vi "NIDCPower_channel_ganging - configure source mode.vi"(8 "error in (no error)":errorcluster, 9 "source mode":T1=1020 items=["Single Point"=1020, "Sequence"=1021], 11 "Ganged Session In":T2) -> (0 "error out":errorcluster, 3 "Ganged Session Out":T2)   [LabVIEW 2021]
uses:
  ctl/NIDCPower_channel_ganging - ctl - ganged config.ctl
  ctl/NIDCPower_channel_ganging - ctl - channel mode.ctl
  ctl/NIDCPower_channel_ganging - ctl - ganged session.ctl
  <instrlib>/niDCPower/nidcpower.llb/niDCPower Source Mode.ctl
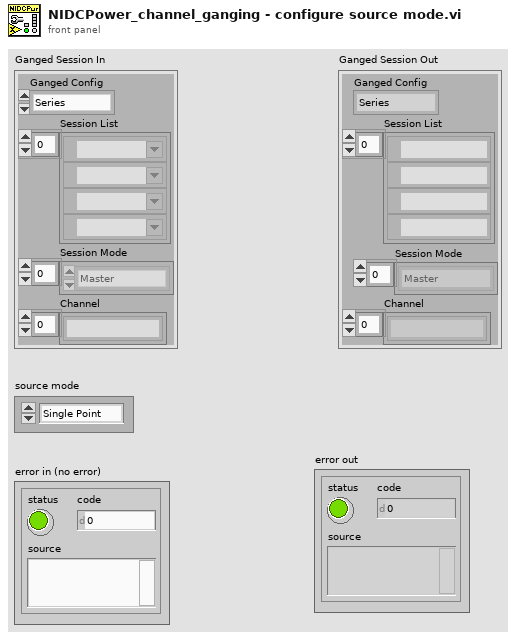
[diagram p1: front panel]
types:
  T1 = typedef "niDCPower Source Mode.ctl" = i32
  T2 = typedef "NIDCPower_channel_ganging - ctl - ganged session.ctl" = cluster{"Ganged Config":T3, "Session List":refnum<k15>[], "Session Mode":T4[], "Channel":string[]}
  T3 = typedef "NIDCPower_channel_ganging - ctl - ganged config.ctl" = enum16{"Series", "Parallel", "Manual"}
  T4 = typedef "NIDCPower_channel_ganging - ctl - channel mode.ctl" = enum16{"Master", "Slave", "Slave - Inverted"}
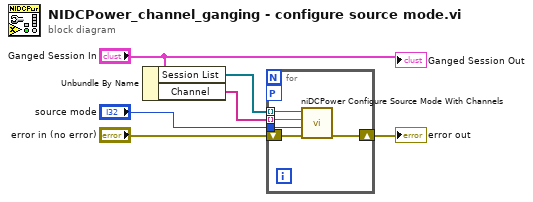
[diagram p0: block diagram]
diagram:
  n1 = Unbundle By Name("Ganged Session In") -> ("Session List"=w6:refnum<k15>[], "Channel"=w1:string[])
  n2 = for {
    workers-P: _ -> [_]
    tunnel: w6 -> [w11] mode=indexing
    tunnel: "source mode" -> [w10]
    shift-right: [w8] -> w2
    shift-left: "error in (no error)" -> [w9]
    tunnel: w1 -> [w7] mode=indexing
    n3 = call <instrlib>:"niDCPower Configure Source Mode With Channels.vi"("error in (no error)"=w9, "source mode"=w10, "channel name"=w7, "instrument handle"=w11) -> ("error out"=w8:errorcluster)  [unwired: 6 in, 1 out]
  }
  "error out" <- w2
  "Ganged Session Out" <- "Ganged Session In"
